vi "Hatch Super Slam Controller.vi"(8 "error in":errorcluster) -> ()   [LabVIEW 2018]
doc: "This VI executes continuously carrying out the current operation and responding to updates or new operations. It will often contain the timing or control code that is difficult to place directly in TeleOp. This VI generally opens all sensors and motors and isolates the rest of the robot code from knowing how the operations are carried out."
uses:
  <vilib>/Rock Robotics/WPI/Framework/Completion Status.ctl
  Hatch Super Slam Setpoints.ctl
  Hatch Super Slam Operations.ctl
  <vilib>/Rock Robotics/WPI/ThirdParty/REV Robotics/SPARK MAX/Typedef/Spark MAX Control Type.ctl
  <vilib>/Rock Robotics/Network Tables/NT Read Boolean.vi
panel:
  out "Encoder value":dbl
  out "Encoder value":dbl(graph)
  out "Squidward's Life Support":dbl
  in  "Interactive Values":T1
  out "Current\nCmd":string
  in  "Buttons":cluster{"Execute Cmd":bool, "Abort Cmd":bool}
  out "Command Timing":cluster{"Start Time (ms)":u32, "Iterations":i32}
  out "Status":T3
  # "Tip: It may be helpful to observe inputs and sensor values.\nYou may also want to display tuning or debugging controls."
  # "Interactive Command: You may fill in the settings for a command\nand schedule it with the Execute button. You can observe and abort\nany command while fine tuning the code for the controller."
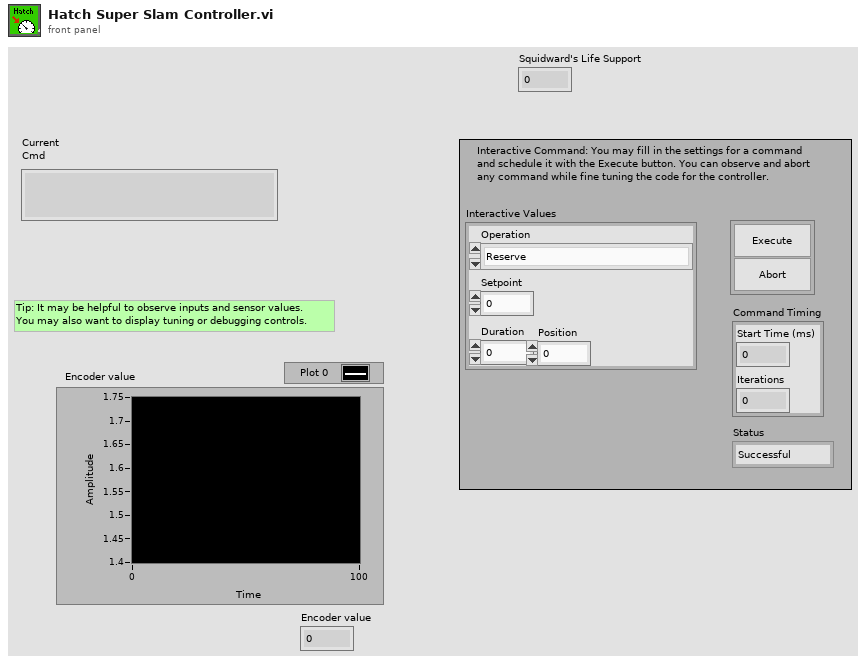
[diagram p1: front panel]
types:
  T1 = typedef "Hatch Super Slam Setpoints.ctl" = cluster{"Operation":T2, "Setpoint":dbl, "Duration":dbl, "Position":dbl}
  T2 = typedef "Hatch Super Slam Operations.ctl" = enum16{"Reserve", "Read Current", "Immediate", "Want to pick up a hatch peice from the ground? Then this super legit super slam subsystem.", "Go To Angle"}
  T3 = typedef "Completion Status.ctl" = enum16{"Successful", "Aborted", "Incomplete"}
  T4 = cluster{"P Gain":dbl, "I Gain":dbl, "D Gain":dbl, "F Gain":dbl, "I Zone":dbl, "Min Output":dbl, "Max Output":dbl}
  T5 = typedef "WPI_MotorControlDeviceRef.ctl" = cluster{"DeviceStatus":errorcluster, "Type":T6, "PWM":cluster{"PWM Channel":T7, "DeadBand":T8}, "CAN":cluster{"Device Number":u8, "SetOutput VI Ref":variant, "GetOutput VI Ref":variant, "Enable VI Ref":variant, "Disable VI Ref":variant, "Data":variant}, "Invert":bool, "DIO PWM":cluster{"PWM \"Enable\" Channel":T7, "DIOChannel":T9, "PWM Rate":dbl}}
  T6 = typedef "WPI_MotorControlType.ctl" = enum16{"PWM", "CAN", "DIO PWM"}
  T7 = typedef "FPGA_DIOPWMChannel.ctl" = enum8{"PWM 0", "PWM 1", "PWM 2", "PWM 3", "PWM 4", "PWM 5", "PWM 6", "PWM 7", "PWM 8", "PWM 9", "PWM MXP 0", "PWM MXP 1", "PWM MXP 2", "PWM MXP 3", "PWM MXP 4", "PWM MXP 5", "PWM MXP 6", "PWM MXP 7", "PWM MXP 8", "PWM MXP 9", "Invalid"}
  T8 = typedef "WPI_PWMDeadband.ctl" = cluster{"Name":string, "maxPositivePwm":i32, "minPositivePwm":i32, "centerPwm":i32, "maxNegativePwm":i32, "minNegativePwm":i32, "angularRange":u16}
  T9 = typedef "FPGA_DIOChannel.ctl" = enum8{"DIO 0", "DIO 1", "DIO 2", "DIO 3", "DIO 4", "DIO 5", "DIO 6", "DIO 7", "DIO 8", "DIO 9", "DIO MXP 0", "DIO MXP 1", "DIO MXP 2", "DIO MXP 3", "DIO MXP 4", "DIO MXP 5", "DIO MXP 6", "DIO MXP 7", "DIO MXP 8", "DIO MXP 9", "DIO MXP 10", "DIO MXP 11", "DIO MXP 12", "DIO MXP 13", "DIO MXP 14", "DIO MXP 15", "SPI Port CS1", "SPI Port CS2", "SPI Port CS3", "SPI Port MISO", "SPI Port MOSI", "Invalid"}
  T10 = typedef "Command Status Info.ctl" = cluster{"Name":string, "Status":T3, "notifier out":T11}
  T11 = typedef "Completion Notifier.ctl" = refnum<notifier>
  T12 = cluster{"Current Command":T1, "Command Timing":cluster{"Start Time (ms)":u32, "Iterations":i32}, "Command Arguments":cluster{"Command Info":T10, "Description":string, "Default Command":T1, "queue out":refnum<queue>, "Subsystem Name":string}}
  T13 = typedef "Spark MAX Control Type.ctl" = enum16{"Percent VBus", "Voltage", "Velocity", "Position", "Smart Motion", "Current", "Smart Velocity"}
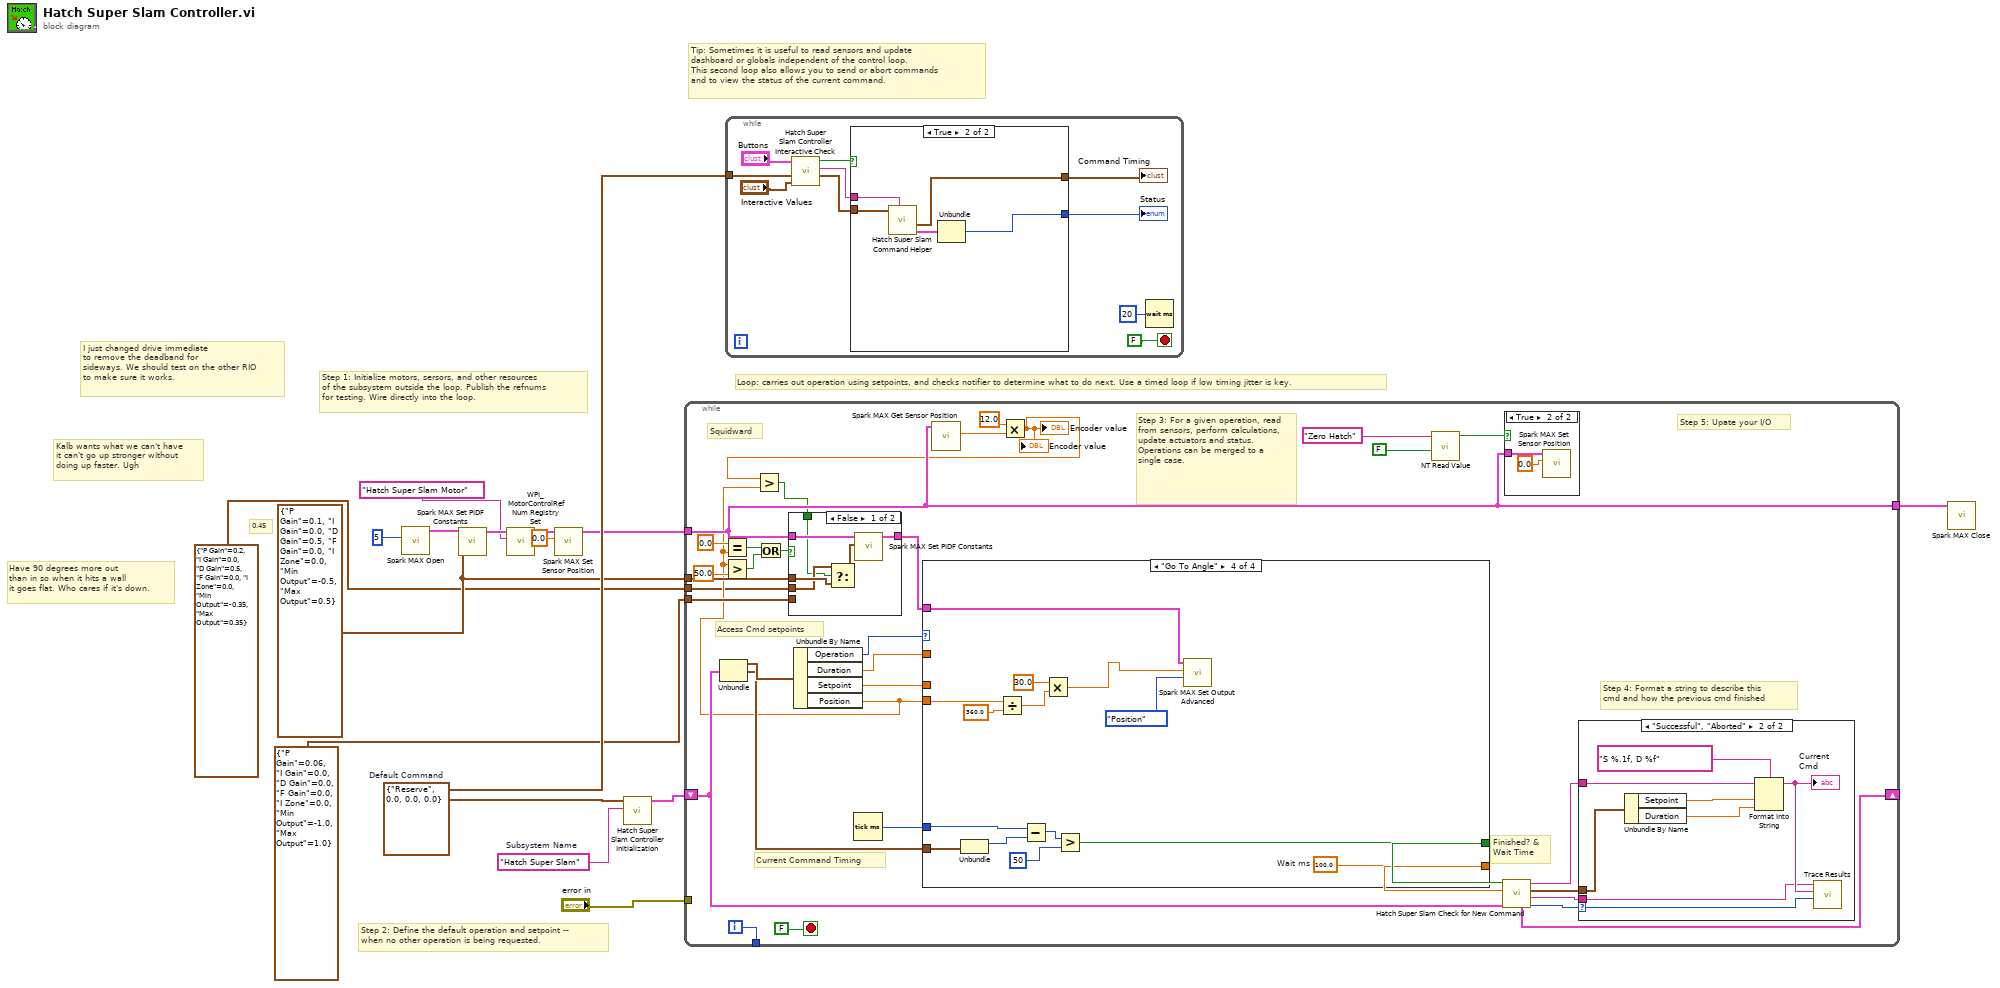
[diagram p0: block diagram]
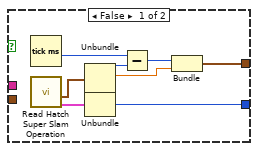
[diagram p2: hidden frame]
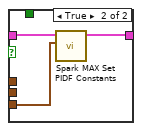
[diagram p3: hidden frame]
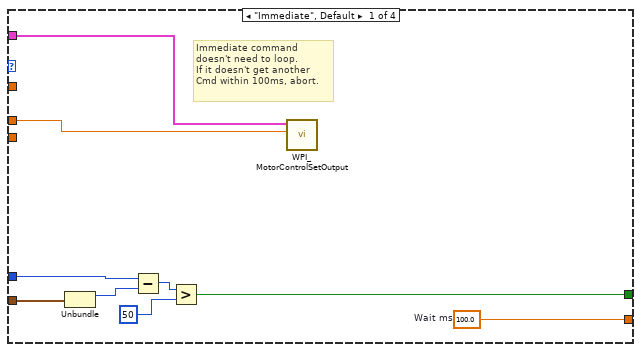
[diagram p6: hidden frame]
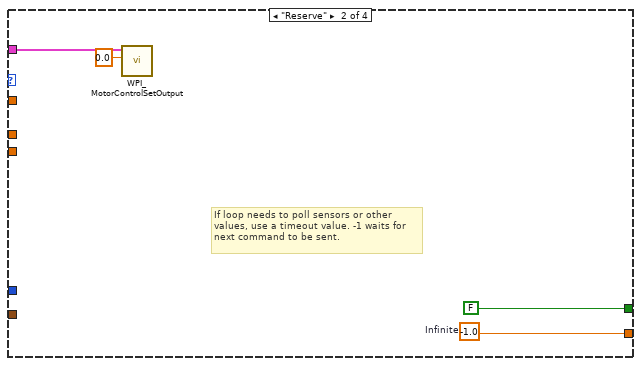
[diagram p7: hidden frame]
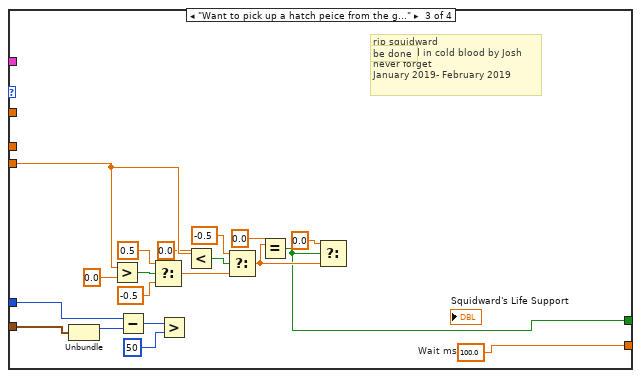
[diagram p8: hidden frame]
diagram:
  w3 = T4 {"P Gain"=0.1, "I Gain"=0.0, "D Gain"=0.5, "F Gain"=0.0, "I Zone"=0.0, "Min Output"=-0.5, "Max Output"=0.5} ("PID Constants")
  w12 = T1 {"Operation"=enum."Reserve", "Setpoint"=0.0, "Duration"=0.0, "Position"=0.0}  # Default Command
  w13 = "Hatch Super Slam"  # Subsystem Name
  # "I just changed drive immediate\nto remove the deadband for\nsideways. We should test on the other RIO\nto make sure it works."
  # "Have 90 degrees more out\nthan in so when it hits a wall\nit goes flat. Who cares if it's down."
  # "Kalb wants what we can't have\nit can't go up stronger without\ndoing up faster. Ugh"
  # "0.45"
  # "Tip: Sometimes it is useful to read sensors and update\ndashboard or globals independent of the control loop.\nThis second loop also allows you to send or abort commands\nand to view the status of the current command."
  # "Step 2: Define the default operation and setpoint --\nwhen no other operation is being requested."
  # "Step 1: Initialize motors, sersors, and other resources\nof the subsystem outside the loop. Publish the refnums\nfor testing. Wire directly into the loop."
  # "Loop: carries out operation using setpoints, and checks notifier to determine what to do next. Use a timed loop if low timing jitter is key."
  n1 = call <vilib>:"Spark MAX Open.vi"("Device Number"=u8 5) -> ("MotorControlDeviceRef"=w10:T5)  [unwired: 9 in, 1 out]
  n2 = call <vilib>:"Spark MAX Set PIDF Constants.vi"("PID Constants"=w3, "MotorControlDeviceRef"=w10) -> ("MotorControlDeviceRef"=w6:T5)  [unwired: 8 in, 1 out]
  n3 = call <vilib>:"WPI_MotorControlRefNum Registry Set.vi"("refnum name"="Hatch Super Slam Motor", "MotorControlDevRef"=w6) -> ("MotorControlDevRef"=w4:T5)  [unwired: 8 in, 1 out]
  n4 = call <vilib>:"Spark MAX Set Sensor Position.vi"("Position"=0.0, "MotorControlDeviceRef"=w4) -> ("MotorControlDeviceRef"=w8:T5)  [unwired: 8 in, 1 out]
  n5 = call "Hatch Super Slam Controller Initialization.vi"("Subsystem Name"=w13, "Default Command"=w12) -> ("Current Command"=w14:T12)  [unwired: 9 in]
  n6 = while {
    shift-right: [w42] -> _
    shift-left: w14 -> [w35]
    tunnel: [w48] -> _
    tunnel: "error in" -> [_]
    tunnel: w8 -> [w27]
    tunnel: [w27] -> w7
    tunnel: w3 -> [w26]
    tunnel: T4 {"P Gain"=0.06, "I Gain"=0.0, "D Gain"=0.0, "F Gain"=0.0, "I Zone"=0.0, "Min Output"=-1.0, "Max Output"=1.0} ("PID Constants") -> [w25]
    tunnel: T4 {"P Gain"=0.2, "I Gain"=0.0, "D Gain"=0.5, "F Gain"=0.0, "I Zone"=0.0, "Min Output"=-0.35, "Max Output"=0.35} ("PID Constants") -> [w17]
    i -> [w48]
    stop <- FALSE stop-if-true
    # "Squidward"
    # "Step 5: Upate your I/O"
    # "Step 4: Format a string to describe this\ncmd and how the previous cmd finished"
    # "Current Command Timing"
    # "Access Cmd setpoints"
    # "Finished? &\nWait Time"
    # "Step 3: For a given operation, read from sensors, perform calculations,\nupdate actuators and status.\nOperations can be merged to a single case."
    n7 = Unbundle(w35) -> ("Current Command"=w47:T1, "Command Timing"=w43:cluster{"Start Time (ms)":u32, "Iterations":i32})  [unwired: 1 out]
    n8 = Unbundle By Name(w47) -> ("Operation"=w46:T2, "Duration"=w45:dbl, "Setpoint"=w34:dbl, "Position"=w19:dbl)
    n9 = Equal?(x=0.0, y=w19) -> (x = y?=w22:bool)
    n10 = Greater?(x=w19, y=50.0) -> (0:w23:bool)
    n11 = Or(x=w22, y=w23) -> (x .or. y?=w24:bool)
    n12 = Tick Count (ms)() -> (millisecond timer value=w44:u32)
    n13 = call <vilib>:"Spark MAX Get Sensor Position.vi"("MotorControlDevRef in"=w27) -> ("Sensor Position"=w29:dbl)  [unwired: 7 in, 3 out]
    n14 = Multiply(x=12.0, y=w29) -> (x*y=w18:dbl)
    "Encoder value" <- w18
    "Encoder value" <- w18
    n15 = Greater?(x=w18, y=w19) -> (0:w16:bool)
    n16 = case shown="False" w24 {
      tunnel: [w55 w58] -> w28
      tunnel: w27 -> [w54 w57]
      tunnel: w26 -> [w53 _]
      tunnel: w25 -> [_ w56]
      tunnel: w17 -> [w51 _]
      tunnel: w16 -> [w50 _]
      frame False {
        n17 = Select(t=w51, s=w50, f=w53) -> (s? t:f=w52:T4)
        n18 = call <vilib>:"Spark MAX Set PIDF Constants.vi"("PID Constants"=w52, "MotorControlDeviceRef"=w54) -> ("MotorControlDeviceRef"=w55:T5)  [unwired: 8 in, 1 out]
      }
      frame True {
        n19 = call <vilib>:"Spark MAX Set PIDF Constants.vi"("PID Constants"=w56, "MotorControlDeviceRef"=w57) -> ("MotorControlDeviceRef"=w58:T5)  [unwired: 8 in, 1 out]
      }
    }
    n20 = case shown="\"Go To Angle\"" w46 {
      tunnel: [w77 w81 w86 w102] -> w40
      tunnel: [w71 FALSE ("ignore previous (F)") w92 w103] -> w41
      tunnel: w43 -> [w73 _ w88 w104]
      tunnel: w45 -> [_ _ _ _]
      tunnel: w44 -> [w72 _ w87 w105]
      tunnel: w19 -> [_ _ w85 w114]
      tunnel: w34 -> [w70 _ _ _]
      tunnel: w28 -> [w69 w79 _ w110]
      frame "Immediate", Default {
        w77 = 100.0  # Wait ms
        # "Immediate command\ndoesn't need to loop.\nIf it doesn't get another\nCmd within 100ms, abort."
        n21 = Unbundle(w73) -> ("Start Time (ms)"=w76:u32)  [unwired: 1 out]
        n22 = Subtract(x=w72, y=w76) -> (x-y=w75:u32)
        n23 = Greater?(x=w75, y=u8 50 ("Left Motor")) -> (0:w71:bool)
        n24 = call <vilib>:"WPI_MotorControlSetOutput.vi"("Output"=w70, "MotorControlDevRef"=w69) -> ()  [unwired: 7 in, 3 out]
      }
      frame "Reserve" {
        w81 = -1.0  # Infinite
        # "If loop needs to poll sensors or other\nvalues, use a timeout value. -1 waits for\nnext command to be sent."
        n25 = call <vilib>:"WPI_MotorControlSetOutput.vi"("Output"=0.0, "MotorControlDevRef"=w79) -> ()  [unwired: 7 in, 3 out]
      }
      frame "Want to pick up a hatch peice from the ground? Then this super legit super slam subsystem." {
        w86 = 100.0  # Wait ms
        # "be done"
        # "rip squidward\nmurdered in cold blood by Josh\nnever forget\nJanuary 2019- February 2019"
        n26 = Unbundle(w88) -> ("Start Time (ms)"=w91:u32)  [unwired: 1 out]
        n27 = Greater?(x=w85, y=0.0) -> (0:w100:bool)
        n28 = Subtract(x=w87, y=w91) -> (x-y=w90:u32)
        n29 = Select(t=0.5, s=w100, f=-0.5) -> (s? t:f=w96:dbl)
        n30 = Greater?(x=w90, y=u8 50 ("Left Motor")) -> ()  [unwired: 1 out]
        n31 = Less?(x=w85, y=0.0) -> (x < y?=w99:bool)
        n32 = Select(t=-0.5, s=w99, f=w96) -> (s? t:f=w93:dbl)
        n33 = Equal?(x=w93, y=0.0) -> (x = y?=w92:bool)
        n34 = Select(t=0.0, s=w92, f=w93) -> ()  [unwired: 1 out]
      }
      frame "Go To Angle" {
        w102 = 100.0  # Wait ms
        n35 = Unbundle(w104) -> ("Start Time (ms)"=w108:u32)  [unwired: 1 out]
        n36 = Divide(x=w114, y=360.0) -> (x/y=w111:dbl)
        n37 = Subtract(x=w105, y=w108) -> (x-y=w107:u32)
        n38 = Multiply(x=30.0, y=w111) -> (x*y=w101:dbl)
        n39 = Greater?(x=w107, y=u8 50 ("Left Motor")) -> (0:w103:bool)
        n40 = call <vilib>:"Spark MAX Set Output Advanced.vi"("Control Mode"=Spark_MAX_Control_Type."Position", "Setpoint"=w101, "MotorControlDevRef"=w110) -> ()  [unwired: 7 in, 2 out]
      }
    }
    n41 = call-poly <vilib>:"NT Read Value.vi"("Default Value"=FALSE, "Name"="Zero Hatch") -> ("Boolean"=w30:bool)  [unwired: 8 in, 1 out]
    n42 = call "Hatch Super Slam Check for New Command.vi"("Current Command"=w35, "Wait time (ms)"=w40, "Finished?"=w41) -> ("Completion"=w36:T3, "Subsystem Name"=w37:string, "Current Command"=w38:T1, "Initial Trace String"=w39:string, "NextCommand"=w42:T12)  [unwired: 4 in]
    n43 = case shown="True" w30 {
      tunnel: w27 -> [_ w59]
      frame False {
      }
      frame True {
        n44 = call <vilib>:"Spark MAX Set Sensor Position.vi"("Position"=0.0, "MotorControlDeviceRef"=w59) -> ()  [unwired: 8 in, 2 out]
      }
    }
    n45 = case shown="\"Successful\", \"Aborted\"" w36 {
      selector: w36 -> [_ w68]
      tunnel: w39 -> [_ w64]
      tunnel: w38 -> [_ w65]
      tunnel: w37 -> [_ w61]
      frame "Incomplete", Default {
        # "Continuing current command"
      }
      frame "Successful", "Aborted" {
        # "Report and setup for next command"
        n46 = Unbundle By Name(w65) -> ("Setpoint"=w67:dbl, "Duration"=w62:dbl)
        n47 = Format Into String(format string="S %.1f, D %f", initial string=w64, w67, w62) -> (resulting string=w63:string)  [unwired: 1 in, 1 out]
        "Current\nCmd" <- w63
        n48 = call <vilib>:"Trace Results.vi"("Status of previous command"=w68, "Description"=w63, "Subsystem"=w61) -> ()  [unwired: 9 in]
      }
    }
  }
  n49 = while {
    tunnel: w12 -> [w121]
    stop <- FALSE stop-if-true
    n50 = call "Hatch Super Slam Controller Interactive Check.vi"("Interactive Command in"="Interactive Values", "Default Command"=w121, "Buttons"="Buttons") -> ("Interactive Command out"=w118:T1, "Trace String"=w119:string, "Schedule"=w120:bool)  [unwired: 6 in]
    n51 = case shown="True" w120 {
      tunnel: [w132 w137] -> w117
      tunnel: w118 -> [_ w135]
      tunnel: [w128 w133] -> w116
      tunnel: w119 -> [_ w136]
      frame False {
        n52 = Tick Count (ms)() -> (millisecond timer value=w127:u32)
        n53 = call "Read Hatch Super Slam Operation.vi"() -> ("Command Info"=w125:T10, "SubSystem Data"=w126:T1)  [unwired: 9 in, 1 out]
        n54 = Unbundle(w126) -> ("Operation"=w131:T2, "Setpoint"=w129:dbl)  [unwired: 2 out]
        n55 = Unbundle(w125) -> ("Status"=w132:T3)  [unwired: 2 out]
        n56 = Subtract(x=w127, y=w131) -> (x-y=w130:u32)
        n57 = Bundle(w130, "Setpoint"=w129) -> (w128:cluster{u32, "Setpoint":dbl})  [unwired: 1 in]
      }
      frame True {
        n58 = call "Hatch Super Slam Command Helper.vi"("Description"=w136, "SubSystem Data"=w135) -> ("Command Info Out"=w134:T10, "Command Timing"=w133:cluster{"Start Time (ms)":u32, "Iterations":i32})  [unwired: 7 in, 1 out]
        n59 = Unbundle(w134) -> ("Status"=w137:T3)  [unwired: 2 out]
      }
    }
    "Status" <- w117
    "Command Timing" <- w116
    n60 = Wait (ms)(milliseconds to wait=u32 20) -> ()  [unwired: 1 out]
  }
  n61 = call <vilib>:"Spark MAX Close.vi"("MotorControlDeviceRef"=w7) -> ()  [unwired: 10 in, 1 out]
